vi "Request Message.vi"(4 "Activate Immediately? (T)":bool=TRUE, 5 "Return Priority (Normal)":T2=enum."Normal", 6 "SubscriptionPolicy":refnum<class "ISubscriptionPolicy.lvclass">, 7 "Desired Notification Msg":refnum<class "Notification Msg.lvclass">, 8 "error in (no error)":errorcluster, 9 "Data Type":variant, 10 "Datum Name":string, 11 "IObserver in":refnum<class "IObserver.lvclass">) -> (0 "error out":errorcluster, 2 "Subscription Policy":T1, 3 "IObserver out":refnum<class "IObserver.lvclass">)   [LabVIEW 2017, in "IObserver.lvlib" / "IObserver.lvclass"]
doc: "<License>\nCopyright © 2017 Composed Systems, LLC | All rights reserved\nwww.composed.io\n\nAuthor: Ethan Stern <ethan.stern@composed.io>\n\nThis software is provided \"AS IS\" WITHOUT WARRANTIES, either express or implied, AND IS FOR EDUCATIONAL PURPOSES ONLY.\n</License>"
uses:
  IObserver.lvclass
  C:/Program Files (x86)/National Instruments/LabVIEW 2017/vi.lib/ActorFramework/Actor/Actor.lvclass
  Transport/ActorMessageTransport/Notification Msg/Notification Msg.lvclass
  <vilib>/ActorFramework/Message Enqueuer/Message Priority.ctl
  IMediator/ISubscriptionPolicy/ISubscriptionPolicy.lvclass
  IMediator/ISubscriptionPolicy/ISubscriptionPolicy Reference.ctl
  <vilib>/ActorFramework/Actor/Actor.lvclass/Actor.ctl
  <vilib>/ActorFramework/Message Enqueuer/Message Enqueuer.lvclass/Message Enqueuer.ctl
  Transport/ActorMessageTransport/ActorMessageTransport.lvclass/ActorMessageTransport.ctl
  IMediator/SubscriptionRequest/SubscriptionRequest.lvclass/SubscriptionRequest.ctl
  IObserver Messages/Subscribe Msg/Subscribe Msg.lvclass/Subscribe Msg.ctl
  <vilib>/ActorFramework/Message Enqueuer/Enqueue.vi
  <vilib>/ActorFramework/Message Enqueuer/Init from Existing Queue.vi
  Transport/ActorMessageTransport/ActorMessageTransport.lvclass
  C:/Git/mva-framework/Framework/IMediator/ITransport/ITransport.lvclass
  IObserver Messages/Subscribe Msg/Subscribe Msg.lvclass
  C:/Program Files (x86)/National Instruments/LabVIEW 2017/vi.lib/ActorFramework/Message/Message.lvclass
  <vilib>/ActorFramework/Message Priority Queue/Priority Enqueue.vi
  Transport/ActorMessageTransport/Notification Msg/Write Notification Msg Return Info.vi
  IMediator/SubscriptionRequest/SubscriptionRequest.lvclass
  <vilib>/ActorFramework/Message Enqueuer/Message Enqueuer.lvclass
  <vilib>/ActorFramework/Actor/Actor.lvclass
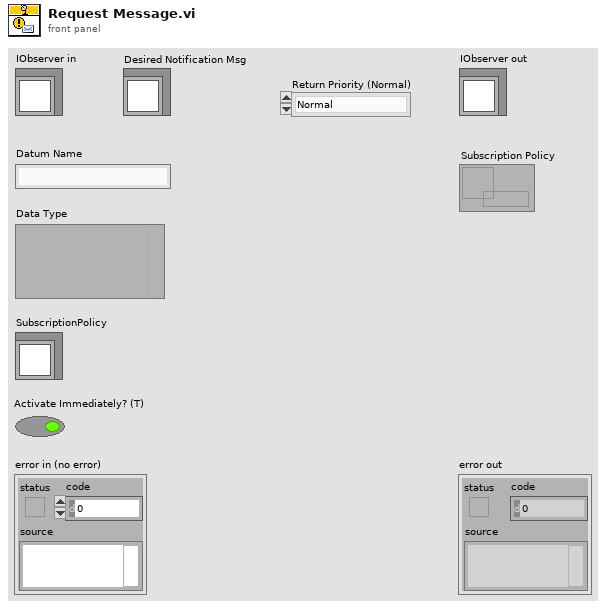
[diagram p1: front panel]
types:
  T1 = typedef "IMediator.lvlib/ISubscriptionPolicy.lvclass/ISubscriptionPolicy Reference.ctl" = refnum<data-value>
  T2 = typedef "Actor Framework.lvlib/Message Enqueuer.lvclass/Message Priority.ctl" = enum16{"Low", "Normal", "High"}
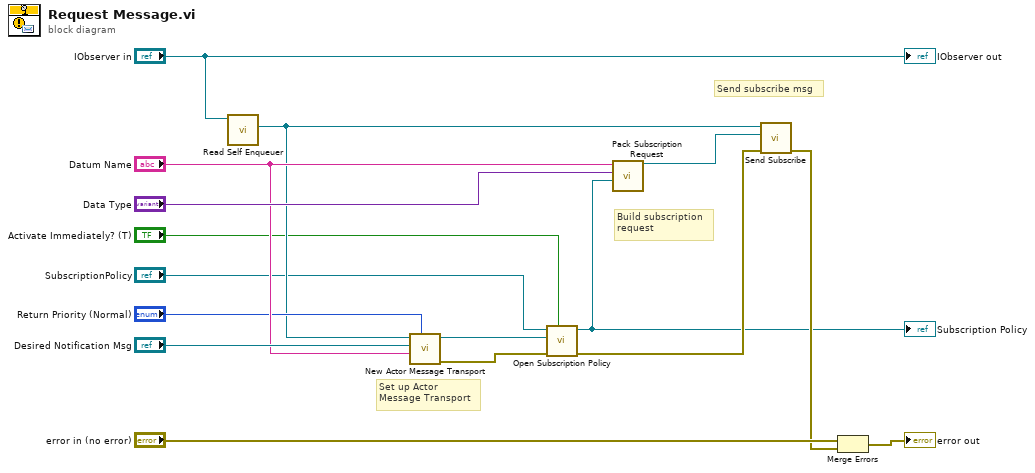
[diagram p0: block diagram]
diagram:
  # "Send subscribe msg"
  # "Build subscription\nrequest"
  # "Set up Actor\nMessage Transport"
  n1 = call <vilib>:"Read Self Enqueuer.vi"("Actor"="IObserver in") -> ("Self Enqueuer"=w6:refnum<class "Message Enqueuer.lvclass">)  [unwired: 10 in]
  n2 = call "New Actor Message Transport.vi"("Return Priority (Normal)"="Return Priority (Normal)", "Datum Name"="Datum Name", "Desired Notification Msg (Type)"="Desired Notification Msg", "Message Enqueuer in"=w6) -> ("error out"=w5:errorcluster, "ActorMessageTransport"=w10:refnum<class "ActorMessageTransport.lvclass">)  [unwired: 6 in]
  n3 = call "Open Subscription Policy.vi"("Activate? (T)"="Activate Immediately? (T)", "error in (no error)"=w5, "Transport"=w10, "SubscriptionPolicy"="SubscriptionPolicy") -> ("error out"=w4:errorcluster, "Subscription Policy"=w3:T1)  [unwired: 6 in]
  "Subscription Policy" <- w3
  n4 = call "Pack Subscription Request.vi"("Subscription Policy"=w3, "Type"="Data Type", "Datum Name"="Datum Name") -> ("SubscriptionRequest"=w15:refnum<class "SubscriptionRequest.lvclass">)  [unwired: 8 in]
  n5 = call "Send Subscribe.vi"("error in (no error)"=w4, "SubscriptionRequest"=w15, "Message Enqueuer"=w6) -> ("error out"=w13:errorcluster)  [unwired: 7 in, 1 out]
  n6 = Merge Errors("error in (no error)", w13) -> (→"error out":errorcluster)
  "IObserver out" <- "IObserver in"
